vi "myVTOL Basic Example.vi"() -> ()   [LabVIEW 2013]
panel:
  in  "Target Sensor Reading":dbl=2.1 step=0.01 format="%#_g V"
  in  "DAQmx Device Name (myDAQ1)":tag="myDAQ1"
  in  "PID Settings":T1={"Proportional"=1.0, "Integral"=0.03, "Derivative"=0.05} {"Derivative" format="%.3f"; "Integral" format="%.2f"; "Proportional" format="%.3f"}
  in  "AutoScale Graph":bool
  out "Sensor Reading":dbl=2.0424252344528213 format="%0.2f V"
  in  "Stop Button":bool
  out "Waveform Chart":cluster{"data":dbl, "Set Point":dbl}(graph)={"data"=2.0424252344528213, "Set Point"=2.1}
  in  "Control Mode":bool
  out "Fan Control Output [V]":dbl(knob)=5.428571428571428 scale=0.0..10.0
  in  "Fan Power Control":dbl(slide)=2.0 scale=0.0..10.0
  # "PITSCO myVTOL - PID Example"
  # "Manual\nFan Power Control"
  # "PID Gain Settings"
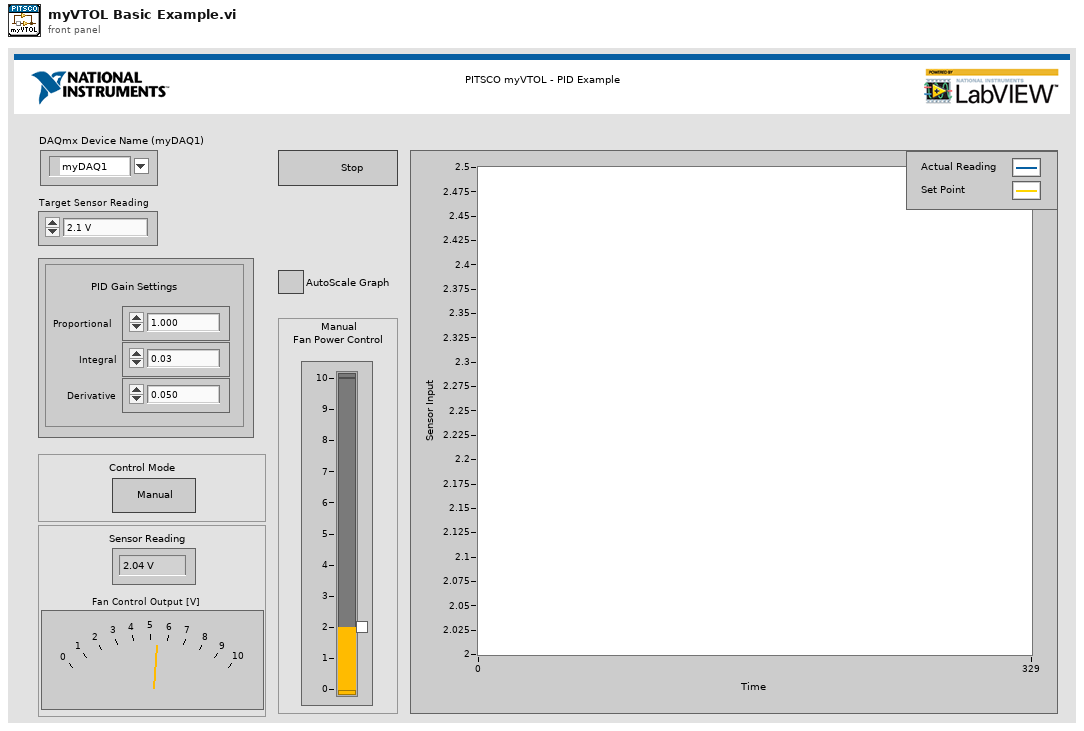
[diagram p1: front panel]
types:
  T1 = cluster{"Proportional":dbl, "Integral":dbl, "Derivative":dbl}
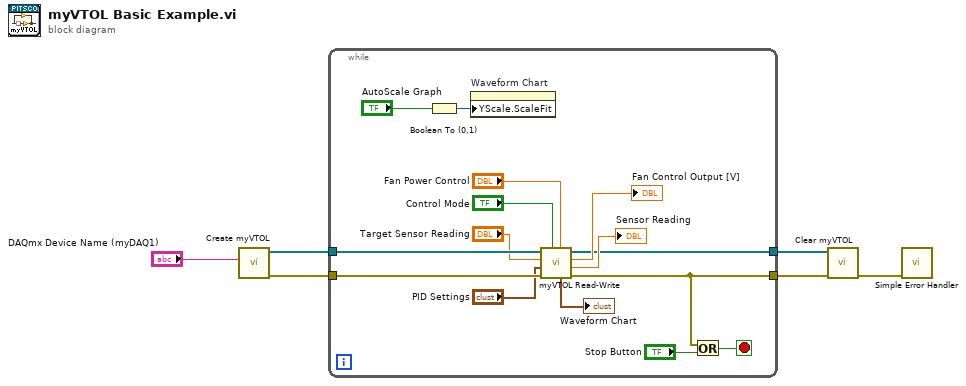
[diagram p0: block diagram]
diagram:
  n1 = call "Create myVTOL.vi"("device name (myDAQ1)"="DAQmx Device Name (myDAQ1)") -> ("error out"=w4:errorcluster, "task array out"=w3:refnum<k21>[])  [unwired: 8 in, 1 out]
  n2 = while {
    tunnel: [w13] -> w6
    tunnel: w4 -> [w21]
    tunnel: w3 -> [w16]
    tunnel: [w7] -> w1
    stop <- w14 stop-if-true
    n3 = Boolean To (0,1)(Boolean="AutoScale Graph") -> (0, 1=w19:i16)
    n4 = property on="Waveform Chart" class="WFChart (strict)"("YScale.ScaleFit"=w19) -> ()  [unwired: 2 in, 2 out]
    n5 = call "myVTOL Read-Write.vi"("Fan Power Control (0V)"="Fan Power Control", "Control Mode (Manual)"="Control Mode", "Error In"=w21, "PID Settings"="PID Settings", "Set Point (2.1V)"="Target Sensor Reading", "task array in"=w16) -> ("Error Out"=w13:errorcluster, "Sensor Reading"=→"Sensor Reading":dbl, "Fan Control Output [V]"=→"Fan Control Output [V]":dbl, "task array out"=w7:refnum<k21>[], "Waveform Chart"=→"Waveform Chart":cluster{"data":dbl, "Set Point":dbl})  [unwired: 1 in]
    n6 = Or(x=w13, y="Stop Button") -> (x .or. y?=w14:bool)
  }
  n7 = call "Clear myVTOL.vi"("Error In"=w6, "task array in"=w1) -> ("Error Out"=w5:errorcluster)  [unwired: 9 in]
  n8 = call <vilib>:"Simple Error Handler.vi"("error in (no error)"=w5) -> ()  [unwired: 4 in, 5 out]
